vi "Get Data From Database.vi"(8 "error in (no error)":errorcluster, 9 "Keyword(\"\")":string, 11 "ScriptDatabase in":refnum<class "ScriptDatabase.lvclass">) -> (0 "error out":errorcluster, 1 "recordset data":variant[][](array[variant]), 3 "Database Out":refnum<class "ScriptDatabase.lvclass">)   [LabVIEW 2015, in "ScriptDatabase.lvclass"]
uses:
  _Database/Implements/ScriptDatabase.lvclass
  _Database/Implements/ScriptDatabase.lvclass/ScriptDatabase.ctl
  _Database/Ancestor/DatabaseAPI.lvclass
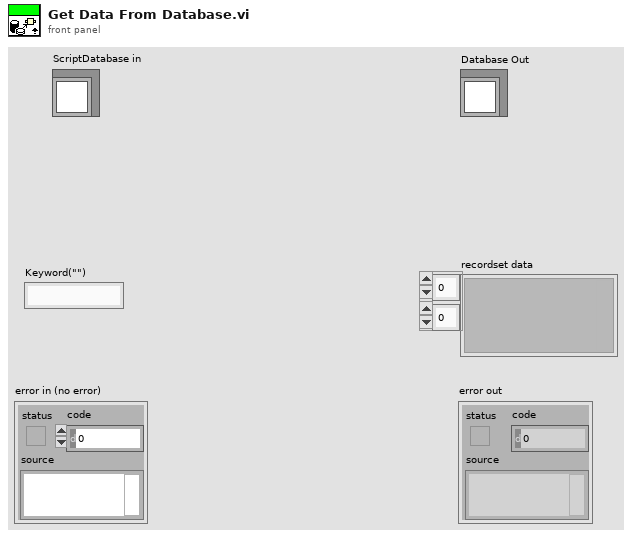
[diagram p1: front panel]
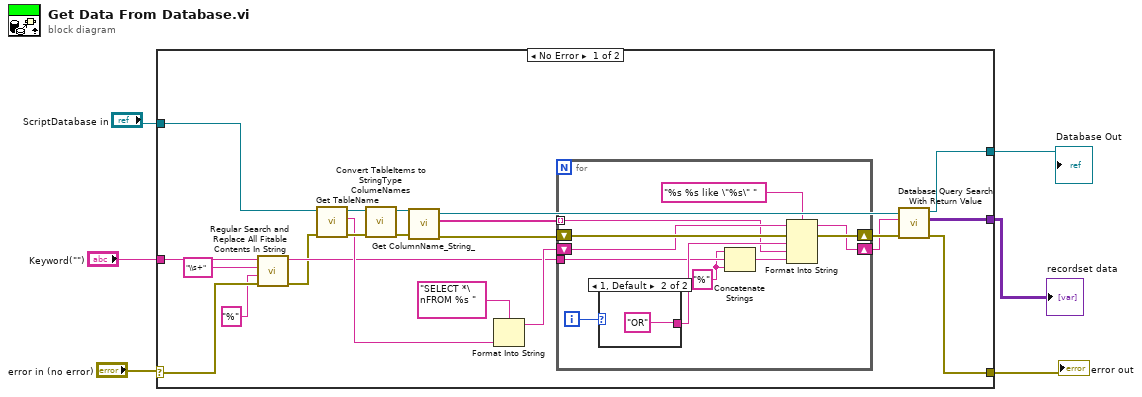
[diagram p0: block diagram]
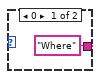
[diagram p2: hidden frame]
diagram:
  n1 = case shown="No Error" "error in (no error)" {
    selector: "error in (no error)" -> [w13 w43]
    tunnel: [w17 w43] -> w4
    tunnel: "Keyword(\"\")" -> [w14 _]
    tunnel: [w15 _] -> w3
    tunnel: "ScriptDatabase in" -> [w8 w42]
    tunnel: [w7 w42] -> w1
    frame No Error {
      n2 = call <userlib>:"Regular Search and Replace All Fitable Contents In String.vi"("error in (no error)"=w13, "replace string (\"\")"="%" ("replace string (\"\")"), "regular expression (\"\")"="\\s+" ("regular expression (\"\")"), "Source(\"\")"=w14) -> ("error out"=w11:errorcluster, "Changed Content(\"\")"=w12:string)  [unwired: 6 in]
      n3 = call "Get TableName.vi"("error in (no error)"=w11, "ScriptDatabase in"=w8) -> ("error out"=w24:errorcluster, "TableName"=w23:string, "ScriptDatabase out"=w25:refnum<class "ScriptDatabase.lvclass">)  [unwired: 7 in]
      n4 = call "Convert TableItems to StringType ColumeNames.vi"("error in (no error)"=w24, "ScriptDatabase in"=w25) -> ("error out"=w21:errorcluster, "ScriptDatabase out"=w22:refnum<class "ScriptDatabase.lvclass">)  [unwired: 8 in]
      n5 = call "Get ColumnName_String_.vi"("error in (no error)"=w21, "ScriptDatabase in"=w22) -> ("error out"=w27:errorcluster, "ColumnName<String>"=w28:string[], "ScriptDatabase out"=w18:refnum<class "ScriptDatabase.lvclass">)  [unwired: 7 in]
      n6 = Format Into String(format string="SELECT *\nFROM %s ", w23) -> (resulting string=w20:string)  [unwired: 2 in, 1 out]
      n7 = for {
        tunnel: w28 -> [w32] mode=indexing
        tunnel: w12 -> [w31]
        shift-right: [w35] -> w19
        shift-left: w27 -> [w36]
        shift-right: [w33] -> w16
        shift-left: w20 -> [w34]
        i -> [w39]
        w29 = "%"
        n8 = case shown="1, Default" w39 {
          tunnel: ["Where" "OR"] -> w37
          frame 0 {
          }
          frame 1, Default {
          }
        }
        n9 = Concatenate Strings(w29, w31, w29) -> (w30:string)
        n10 = Format Into String(format string="%s %s like \"%s\" ", initial string=w34, error in=w36, w37, w32, w30) -> (resulting string=w33:string, error out=w35:errorcluster)
      }
      n11 = call "Database Query Search With Return Value.vi"("error in (no error)"=w19, "SQL query"=w16, "object in"=w18) -> ("error out"=w17:errorcluster, "recordset data"=w15:variant[][], "object out"=w7:refnum<class "ScriptDatabase.lvclass">)  [unwired: 5 in, 1 out]
    }
    frame Error {
    }
  }
  "error out" <- w4
  "recordset data" <- w3
  "Database Out" <- w1
